vi "Setting Database.GetPublicEvents.vi"(8 "error in (no error)":errorcluster, 11 "Setting Database":refnum<class "Setting Database.lvclass">) -> (0 "error out":errorcluster, 2 "Public Events":T1, 3 "Setting Database out":refnum<class "Setting Database.lvclass">)   [LabVIEW 2019, in "Setting Database.lvclass"]
doc: "---------------------------------------------------------------\nJKI State Machine Objects™\nhttp://jki.net/state-machine-objects/\nCopyright (C) 2005-2015, JKI <info@jki.net>\nALL RIGHTS RESERVEDJKI State Machine Objects (SMO) 1.0.0.4\nJKI - JKI\nCopyright (c) 2015, JKI"
uses:
  Setting Database.lvclass
  Typedefs/PublicEvents--Cluster.ctl
  Typedefs/PublicEvents--Setting Database.NewActivePath.ctl
  Path Settings/Path Settings.lvclass
  Typedefs/PublicEvents--Setting Database.PathsUpdatedCheck.ctl
  Typedefs/PublicEvents--Setting Database.PathsUpdated.ctl
  Typedefs/PublicEvents--Setting Database.RectanglesUpdatedCheck.ctl
  Typedefs/PublicEvents--Setting Database.RectanglesUpdated.ctl
  Rectangle Settings/Rectangle Settings.lvclass
  Typedefs/PublicEvents--Setting Database.NewActiveRectangle.ctl
  Typedefs/PublicEvents--Setting Database.NewActiveFunnel.ctl
  Funnel Settings/Funnel Settings.lvclass
  Typedefs/PublicEvents--Setting Database.FunnelsUpdatedCheck.ctl
  Typedefs/PublicEvents--Setting Database.FunnelsUpdated.ctl
  Typedefs/PublicEvents--Setting Database.NewActiveDot.ctl
  Dot Settings/Dot Settings.lvclass
  Typedefs/PublicEvents--Setting Database.DotsUpdatedCheck.ctl
  Typedefs/PublicEvents--Setting Database.DotsUpdated.ctl
  Setting Database.lvclass/Setting Database.ctl
panel:
  # "For instructions on how to use the JKI State Machine Objects, examples and video tutorials, visit:\nhttp://jki.net/state-machine-objects/\n\nJKI State Machine Objects™\nhttp://jki.net/state-machine-objects/\nCopyright (C) 2005-2015, JKI <info@jki.net>\nALL RIGHTS RESERVED"
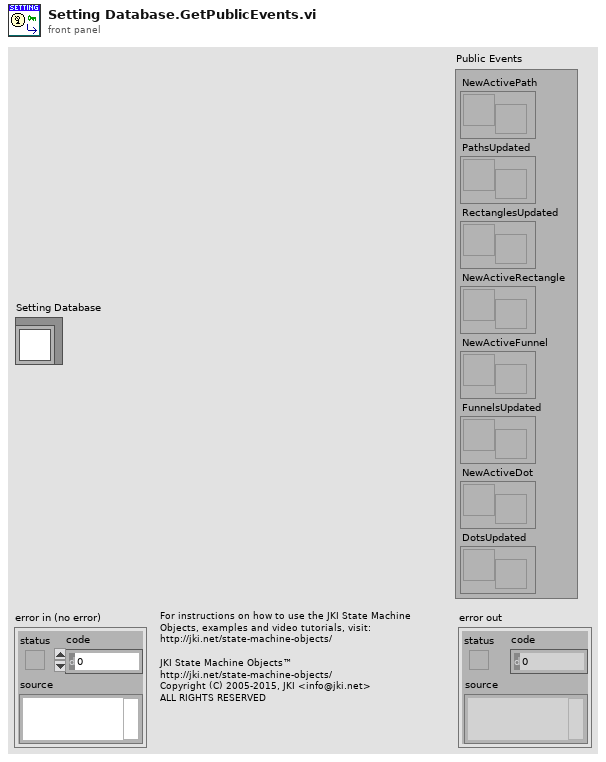
[diagram p1: front panel]
types:
  T1 = typedef "Setting Database.lvclass/PublicEvents--Cluster.ctl" = cluster{"NewActivePath":refnum<user-event>, "PathsUpdated":refnum<user-event>, "RectanglesUpdated":refnum<user-event>, "NewActiveRectangle":refnum<user-event>, "NewActiveFunnel":refnum<user-event>, "FunnelsUpdated":refnum<user-event>, "NewActiveDot":refnum<user-event>, "DotsUpdated":refnum<user-event>}
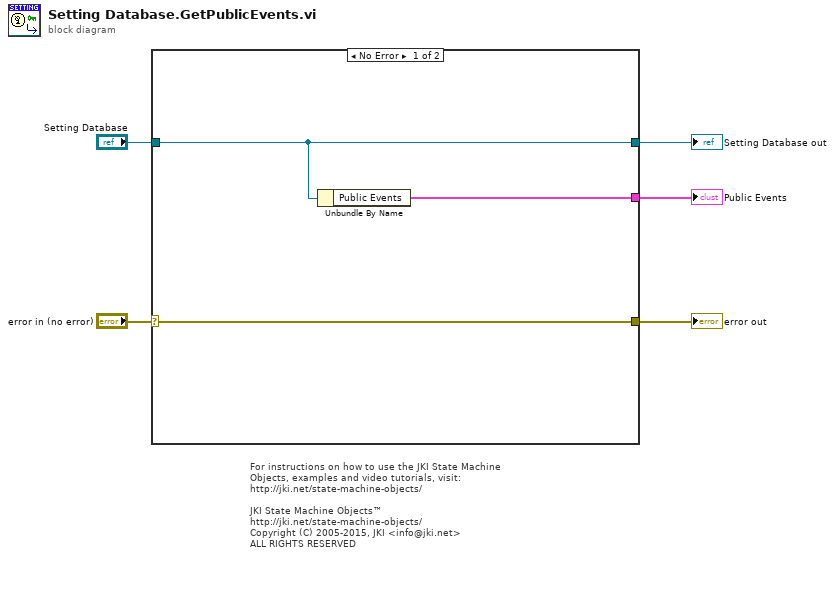
[diagram p0: block diagram]
diagram:
  # "For instructions on how to use the JKI State Machine Objects, examples and video tutorials, visit:\nhttp://jki.net/state-machine-objects/\n\nJKI State Machine Objects™\nhttp://jki.net/state-machine-objects/\nCopyright (C) 2005-2015, JKI <info@jki.net>\nALL RIGHTS RESERVED"
  n1 = case shown="No Error" "error in (no error)" {
    selector: "error in (no error)" -> [w7 w9]
    tunnel: "Setting Database" -> [w6 w10]
    tunnel: [w7 w9] -> w4
    tunnel: [w6 w10] -> w3
    tunnel: [w8 _] -> w1
    frame No Error {
      n2 = Unbundle By Name(w6) -> ("Public Events"=w8:T1)
    }
    frame Error {
    }
  }
  "error out" <- w4
  "Setting Database out" <- w3
  "Public Events" <- w1
